vi "smaract serial read positions.vi"(8 "error in (no error)":errorcluster, 11 "VISA Refnum in":refnum<visa-resource-name>) -> (0 "error out":errorcluster, 1 "Positions":i32[](array[numeric]), 2 "Get position commands":string[](array[string]), 3 "VISA Refnum out":refnum<visa-resource-name>)   [LabVIEW 2020, in "Smaract.lvclass"]
uses:
  Smaract.lvclass
  shared/stop FGV control.ctl
  smaract serial read hardware part.vi
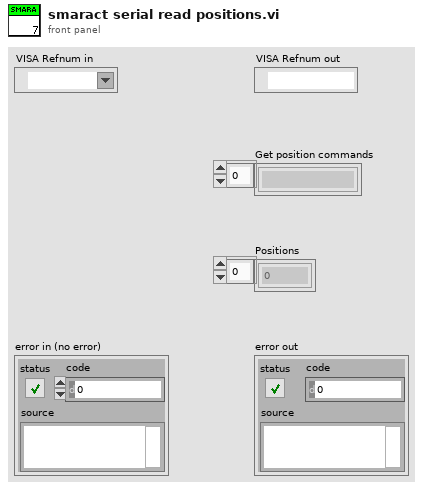
[diagram p1: front panel]
types:
  T1 = typedef "stop FGV control.ctl" = enum16{"Clear", "Write", "Read"}
  T2 = typedef "Smaract acquire fgv.ctl" = cluster{"busy":bool, "Positions":i32[]}
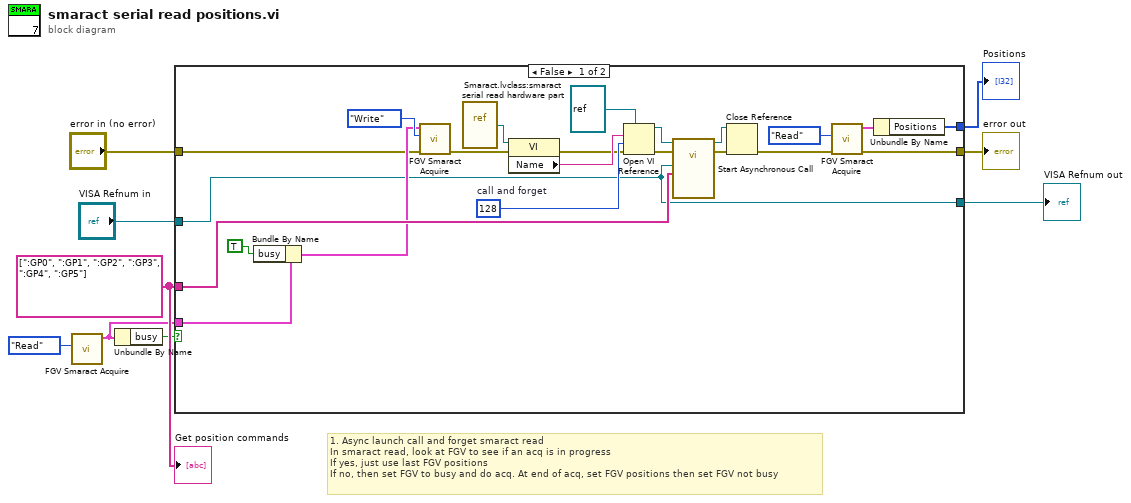
[diagram p0: block diagram]
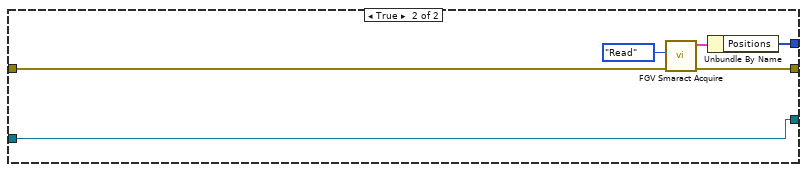
[diagram p2: hidden frame]
diagram:
  w4 = string[] [":GP0", ":GP1", ":GP2", ":GP3", ":GP4", ":GP5"]
  # "1. Async launch call and forget smaract read\nIn smaract read, look at FGV to see if an acq is in progress\nIf yes, just use last FGV positions\nIf no, then set FGV to busy and do acq. At end of acq, set FGV positions then set FGV not busy"
  n1 = call "FGV Smaract Acquire.vi"("Function"=stop_FGV_control."Read") -> ("Smaract Acq Data 2"=w1:T2)  [unwired: 9 in, 1 out]
  n2 = Unbundle By Name(w1) -> ("busy"=w2:bool)
  n3 = case shown="False" w2 {
    tunnel: [w15 w37] -> w9
    tunnel: [w10 w34] -> w8
    tunnel: [w11 w32] -> w7
    tunnel: "VISA Refnum in" -> [w15 w37]
    tunnel: "error in (no error)" -> [w17 w33]
    tunnel: w4 -> [w22 _]
    tunnel: w1 -> [w20 _]
    frame False {
      w31 = 128  # call and forget
      n4 = Bundle By Name(cluster=w20, "busy"=TRUE) -> (w18:T2)
      n5 = call "FGV Smaract Acquire.vi"("error in"=w17, "Function"=stop_FGV_control."Write", "Smaract Acq Data"=w18) -> ("error out"=w16:errorcluster)  [unwired: 7 in, 1 out]
      n6 = vi-ref "Smaract.lvclass:smaract serial read hardware part.vi"() -> (w23:refnum<vi>)
      n7 = property class="VI"(reference=w23, error in=w16) -> (error out=w24:errorcluster, "Name"=w25:string)  [unwired: 1 out]
      n8 = Open VI Reference(type specifier VI Refnum (for type only)=refnum<vi> refnum, vi path=w25, options=w31, error in (no error)=w24) -> (vi reference=w29:refnum<vi>, error out=w28:errorcluster)  [unwired: 2 in]
      n9 = call-by-ref "Start Asynchronous Call"(reference=w29, error in=w28, "Array in"=w22, "VISA Refnum in"=w15) -> (reference out=w26:refnum<vi>, error out=w27:errorcluster)  [unwired: 7 in, 3 out]
      n10 = Close Reference(reference=w26, error in (no error)=w27) -> (error out=w12:errorcluster)
      n11 = call "FGV Smaract Acquire.vi"("error in"=w12, "Function"=stop_FGV_control."Read") -> ("error out"=w11:errorcluster, "Smaract Acq Data 2"=w13:T2)  [unwired: 8 in]
      n12 = Unbundle By Name(w13) -> ("Positions"=w10:i32[])
    }
    frame True {
      n13 = call "FGV Smaract Acquire.vi"("error in"=w33, "Function"=stop_FGV_control."Read") -> ("error out"=w32:errorcluster, "Smaract Acq Data 2"=w35:T2)  [unwired: 8 in]
      n14 = Unbundle By Name(w35) -> ("Positions"=w34:i32[])
    }
  }
  "VISA Refnum out" <- w9
  "Positions" <- w8
  "error out" <- w7
  "Get position commands" <- w4
